vi "IO@Exchange__Parameter.vi"(1 "ParamterIn":string) -> (0 "ParamterOut":string)   [LabVIEW 2020]
panel:
  in  "IO2":string(combo)="On"
  in  "IO1":string(combo)
  in  "Confirm":bool
  # "IO@Exchange $IO1,$IO2"
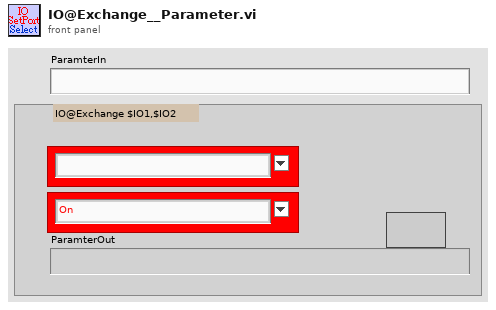
[diagram p1: front panel]
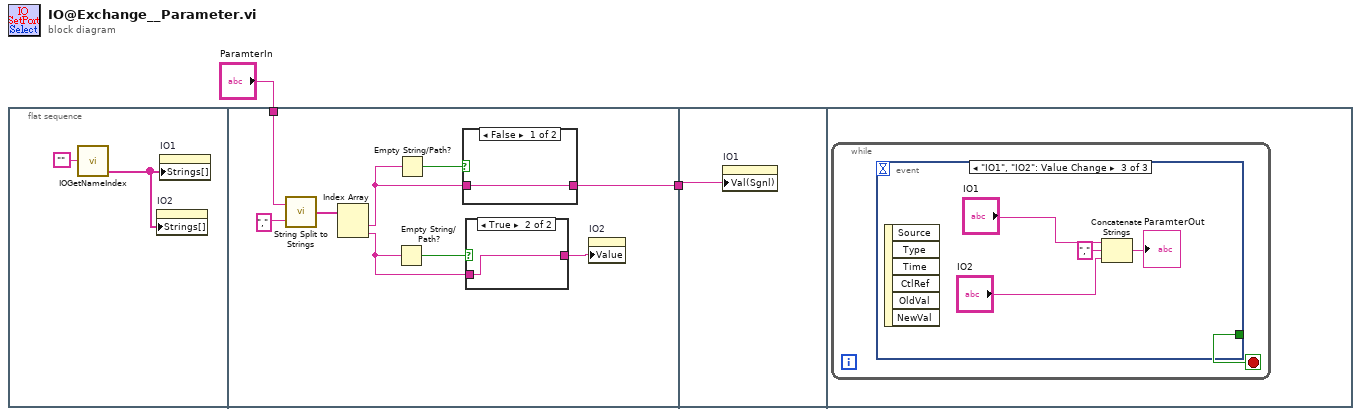
[diagram p0: block diagram]
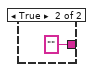
[diagram p3: hidden frame]
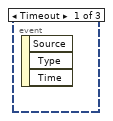
[diagram p4: hidden frame]
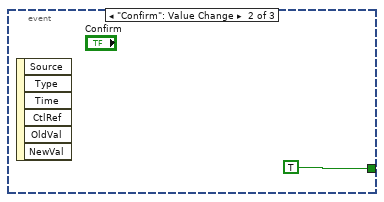
[diagram p5: hidden frame]
diagram:
  n1 = flat-sequence {
    tunnel: "ParamterIn" -> [w12]
    tunnel: [w5] -> w1
    tunnel: w1 -> [w18]
    frame #0 {
      n2 = call "IOGetNameIndex.vi"("PortName"="") -> ("PortNameList Out"=w3:string[])  [unwired: 3 in, 1 out]
      n3 = property on="IO2" class="CmbBox"("Strings[]"=w3) -> ()  [unwired: 2 in, 2 out]
      n4 = property on="IO1" class="CmbBox"("Strings[]"=w3) -> ()  [unwired: 2 in, 2 out]
    }
    frame #1 {
      n5 = call "String Split to Strings.vi"("search string/char (-)"=",", "String"=w12) -> ("Array"=w11:string[])
      n6 = Index Array(array=w11) -> (element #1=w9:string, element #2=w7:string)  [unwired: 2 in]
      n7 = Empty String/Path?(string/path=w7) -> (empty?=w8:bool)
      n8 = Empty String/Path?(string/path=w9) -> (empty?=w10:bool)
      n9 = case shown="False" w10 {
        tunnel: w9 -> [w16 _]
        tunnel: [w16 ""] -> w5
        frame False {
        }
        frame True {
        }
      }
      n10 = case shown="True" w8 {
        tunnel: w7 -> [w14 w15]
        tunnel: [w14 w15] -> w6
        frame False {
        }
        frame True {
        }
      }
      n11 = property on="IO2" class="CmbBox"("Value"=w6) -> ()  [unwired: 2 in, 2 out]
    }
    frame #2 {
      n12 = property on="IO1" class="CmbBox"("Val(Sgnl)"=w18) -> ()  [unwired: 2 in, 2 out]
    }
    frame #3 {
      n13 = while {
        stop <- w19 stop-if-true
        n14 = event shown="[2] \"IO1\", \"IO2\": Value Change" {
          selector: _ -> [_ _ _]
          dyn-events: _ -> [_ _ _]
          timeout: _ -> [_ _ _]
          tunnel: [_ TRUE _] -> w19
          event Timeout {
            n15 = event-data() -> ()  [unwired: 1 in, 3 out]
          }
          event "Confirm": Value Change {
            n16 = event-data() -> ()  [unwired: 1 in, 6 out]
          }
          event "IO1", "IO2": Value Change {
            n17 = event-data() -> ()  [unwired: 1 in, 6 out]
            n18 = Concatenate Strings("IO1", "," ("string"), "IO2") -> (→"ParamterOut":string)
          }
        }
      }
    }
  }
